vi "Handle Command.vi"(8 "error in (no error)":errorcluster, 9 "params in":variant, 10 "command":string, 11 "Instrument.Framework-Template in":refnum<class "Instrument.Framework-Template.lvclass">) -> (0 "error out":errorcluster, 1 "processed data":variant, 2 "command out":string, 3 "Instrument.Framework-Template out":refnum<class "Instrument.Framework-Template.lvclass">)   [LabVIEW 2019, in "Instrument.Framework-Template.lvclass"]
uses:
  Instrument.Framework-Template.lvclass
  Typedefs/Instrument.Framework-Template.Commands--Enum.ctl
  Instrument.Framework-Template.lvclass/Instrument.Framework-Template.ctl
  7d5c8d57-f0a0-4908-8abf-1b878744cce4.vi
  7d5c8d57-f0a0-4908-8abf-1b878744cce4.vi/27d2e435-2ae7-4c33-9f07-3c99efbda6af.vi
  7d5c8d57-f0a0-4908-8abf-1b878744cce4.vi/22d6071b-4a01-470b-84c6-ee3bdff3db2c.vi
  <vilib>/Utility/Data Type/Get Type Information.vi
  <vilib>/JDP Science/JSONtext/JSON text to Variant.vi
  <vilib>/JDP Science/JSONtext/LVClass Serializer/JSONtext LVClass Serializer.lvclass
  Framework/Instrument Types/SCPI/Instrument.SCPI.lvclass
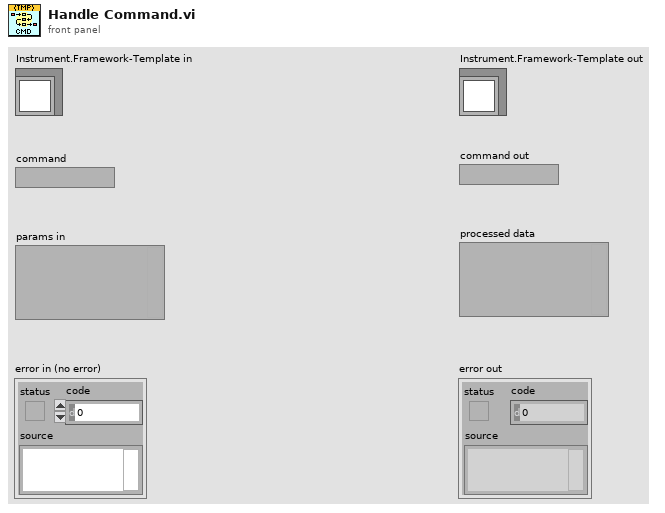
[diagram p1: front panel]
types:
  T1 = typedef "Instrument.Framework-Template.lvclass/Instrument.Framework-Template.Commands--Enum.ctl" = enum16{"doSomething"}
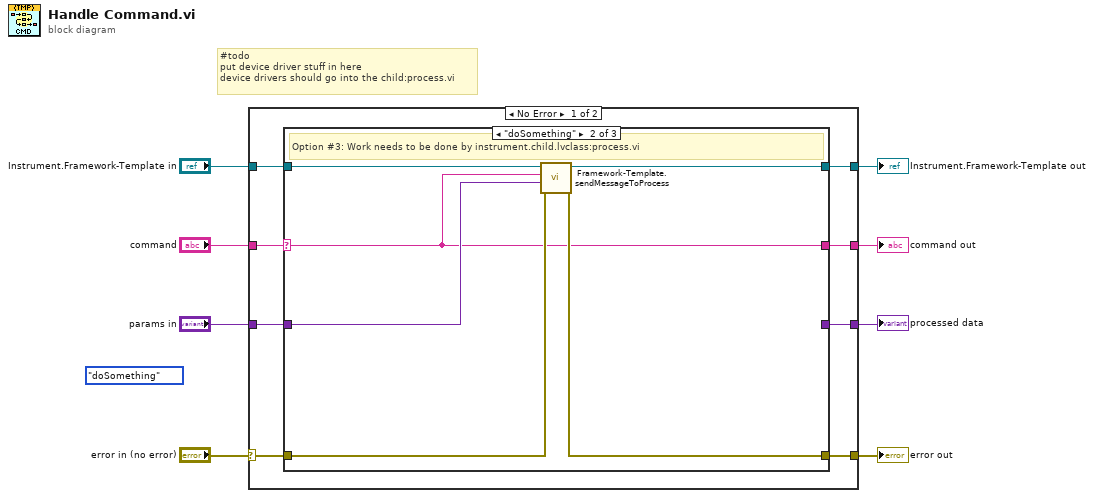
[diagram p0: block diagram]
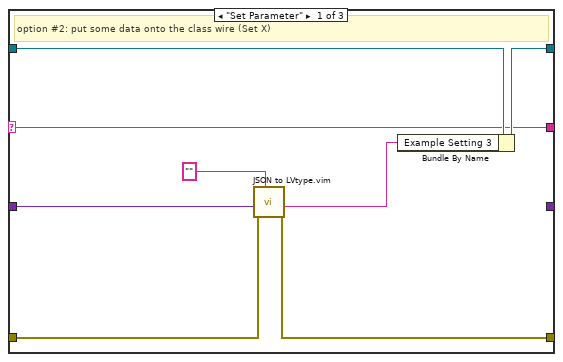
[diagram p2: hidden frame]
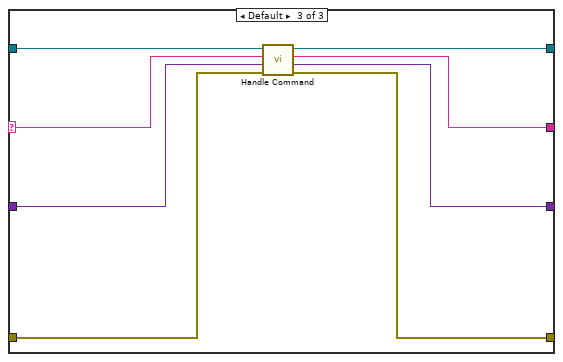
[diagram p3: hidden frame]
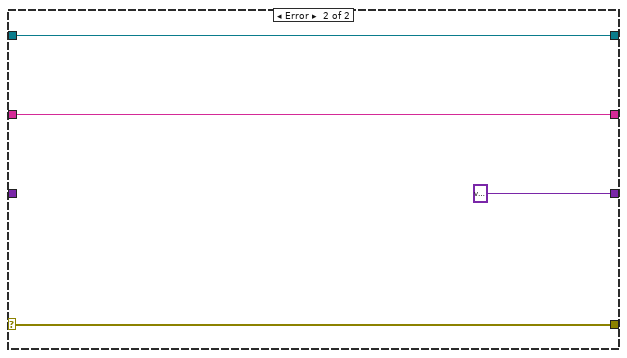
[diagram p4: hidden frame]
diagram:
  (unwired) Instrument.Framework-Template.Commands--Enum."doSomething" ("Commands")
  # "#todo\nput device driver stuff in here\ndevice drivers should go into the child:process.vi"
  n1 = case shown="No Error" "error in (no error)" {
    selector: "error in (no error)" -> [w10 w42]
    tunnel: [w12 w42] -> w6
    tunnel: [w14 w41] -> w5
    tunnel: "Instrument.Framework-Template in" -> [w15 w41]
    tunnel: "command" -> [w16 w40]
    tunnel: [w13 variant ("Variant")] -> w3
    tunnel: "params in" -> [w9 _]
    tunnel: [w11 w40] -> w1
    frame No Error {
      n2 = case shown="\"doSomething\"" w16 {
        selector: w16 -> [w19 w25 w32]
        tunnel: w15 -> [w24 w30 w36]
        tunnel: [w23 w29 w33] -> w14
        tunnel: [_ _ w35] -> w13
        tunnel: w10 -> [w22 w28 w37]
        tunnel: w9 -> [w20 w26 w38]
        tunnel: [w21 w27 w34] -> w12
        tunnel: [w19 w25 w31] -> w11
        frame "Set Parameter" {
          # "option #2: put some data onto the class wire (Set X)"
          n3 = call "JSON to LVtype.vim"("type"="", "error in (no error)"=w22, "JSON Data in"=w20) -> ("error out"=w21:errorcluster, "Data out"=w18:string)  [unwired: 7 in]
          n4 = Bundle By Name(cluster=w24, "Example Setting 3"=w18) -> (w23:refnum<class "Instrument.Framework-Template.lvclass">)
        }
        frame "doSomething" {
          # "Option #3: Work needs to be done by instrument.child.lvclass:process.vi"
          n5 = call "Framework-Template.sendMessageToProcess.vi"("error in (no error)"=w28, "Data"=w26, "Command"=w25, "Framework-Template in"=w30) -> ("error out"=w27:errorcluster, "Framework-Template out"=w29:refnum<class "Instrument.Framework-Template.lvclass">)  [unwired: 6 in]
        }
        frame Default {
          n6 = call-parent "Handle Command.vi"("error in (no error)"=w37, "params in"=w38, "command"=w32, "Instrument in"=w36) -> ("error out"=w34:errorcluster, "processed data"=w35:variant, "command out"=w31:string, "Instrument out"=w33:refnum<class "Instrument.Framework-Template.lvclass">)  [unwired: 4 in]
        }
      }
    }
    frame Error {
    }
  }
  "error out" <- w6
  "Instrument.Framework-Template out" <- w5
  "command out" <- w1
  "processed data" <- w3
